vi "Update Index.vi"(8 "error in (no error)":errorcluster, 10 "Index":i32, 11 "Team Config Panel in":refnum<class "Team Config Panel.lvclass">) -> (0 "error out":errorcluster, 3 "Team Config Panel out":refnum<class "Team Config Panel.lvclass">)   [LabVIEW 2020, in "SB App.lvlib" / "Team Config Panel.lvclass"]
uses:
  Team Config Panel.lvclass
  Team Index Data.ctl
  Team Config Panel.lvclass/Team Config Panel.ctl
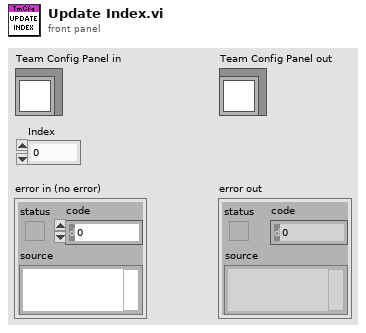
[diagram p1: front panel]
types:
  T1 = typedef "SB App.lvlib/Team Config Panel.lvclass/Team Index Data.ctl" = cluster{"Team Index":i32}
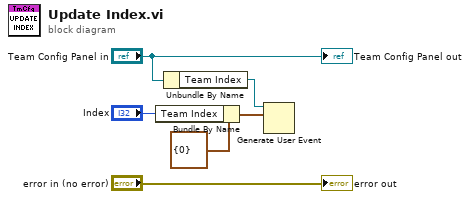
[diagram p0: block diagram]
diagram:
  n1 = Bundle By Name(cluster=T1 {"Team Index"=0} ("event data"), "Team Index"="Index") -> (w2:T1)
  n2 = Unbundle By Name("Team Config Panel in") -> ("Team Index"=w4:refnum<user-event>)
  n3 = Generate User Event(user event=w4, event data cluster=w2) -> ()  [unwired: 2 in, 2 out]
  "error out" <- "error in (no error)"
  "Team Config Panel out" <- "Team Config Panel in"
